vi "uPython_Close.vi"(8 "error in":errorcluster, 11 "VISA  in":refnum<visa-resource-name>) -> (0 "error out":errorcluster, 3 "VISA  out":refnum<visa-resource-name>)   [LabVIEW 2016]
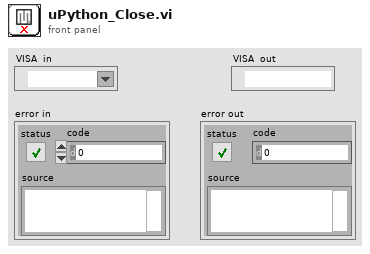
[diagram p1: front panel]
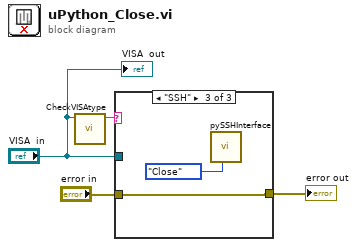
[diagram p0: block diagram]
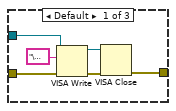
[diagram p2: hidden frame]
diagram:
  n1 = call "CheckVISAtype.vi"("VISA Refnum in"="VISA  in") -> ("data string"=w1:string)  [unwired: 9 in, 1 out]
  n2 = case shown="\"SSH\"" w1 {
    tunnel: [w10 w11 w13] -> w4
    tunnel: "error in" -> [w9 w11 w13]
    tunnel: "VISA  in" -> [w8 _ _]
    frame Default {
      n3 = VISA Write(VISA resource name=w8, write buffer="\u0003", error in (no error)=w9) -> (VISA resource name out=w7:refnum<visa-resource-name>, error out=w6:errorcluster)  [unwired: 1 out]
      n4 = VISA Close(VISA resource name=w7, error in (no error)=w6) -> (error out=w10:errorcluster)
    }
    frame "" {
    }
    frame "SSH" {
      n5 = call "pySSHInterface.vi"("Task"=enum16{"Init", "Read", "Write", "Close"}."Close") -> ()  [unwired: 10 in, 1 out]
    }
  }
  "error out" <- w4
  "VISA  out" <- "VISA  in"
